vi "Update Linkage Table Items.vi"(8 "error in (no error)":errorcluster, 10 "Variables":string[](array[string]), 11 "Item Names":string[][](array[string])) -> (0 "error out":errorcluster, 3 "Item Names":string[][](array[string]))   [LabVIEW 2019, in "Instrument Addon System Explorer.lvlib"]
uses:
  Instrument Addon System Explorer.lvlib
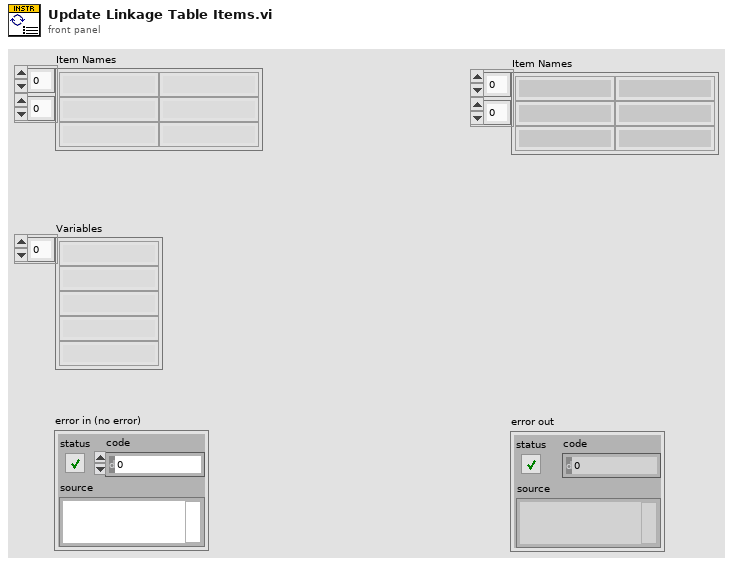
[diagram p1: front panel]
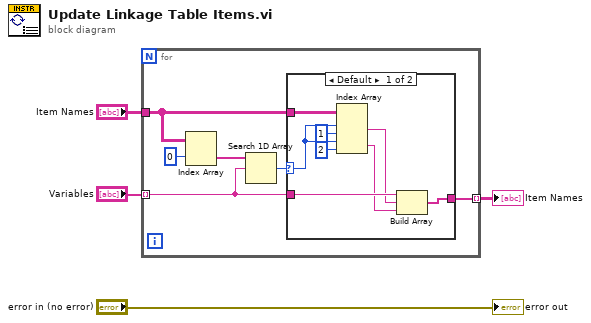
[diagram p0: block diagram]
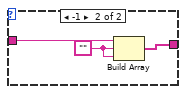
[diagram p2: hidden frame]
diagram:
  n1 = for {
    tunnel: "Variables" -> [w9] mode=indexing
    tunnel: "Item Names" -> [w6]
    tunnel: [w8] -> w2 mode=indexing
    n2 = Index Array(array=w6, index (col)=0 ("disabled index (col)")) -> (element=w7:string[])  [unwired: 1 in]
    n3 = Search 1D Array(1D array=w7, element=w9) -> (index of element=w10:i32)  [unwired: 1 in]
    n4 = case shown="Default" w10 {
      selector: w10 -> [w13 _]
      tunnel: w9 -> [w18 w21]
      tunnel: [w15 w20] -> w8
      tunnel: w6 -> [w17 _]
      frame Default {
        n5 = Index Array(array=w17, index (row) #1=w13, index (col) #1=1 ("disabled index (col)"), index (row) #2=w13, index (col) #2=2 ("disabled index (col)")) -> (element #1=w16:string, element #2=w11:string)
        n6 = Build Array(w18, w16, w11) -> (w15:string[])
      }
      frame -1 {
        w19 = ""
        n7 = Build Array(w21, w19, w19) -> (w20:string[])
      }
    }
  }
  "Item Names" <- w2
  "error out" <- "error in (no error)"
